vi "ex32.vi"(11 "Data":string) -> ()   [LabVIEW 2019]
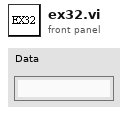
[diagram p1: front panel]
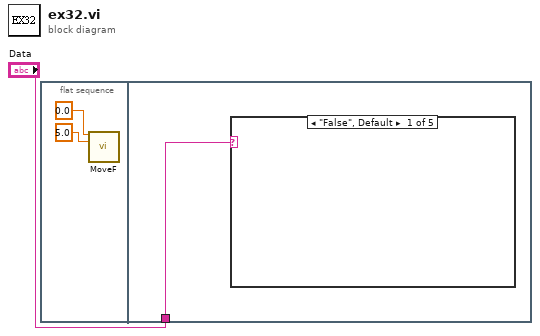
[diagram p0: block diagram]
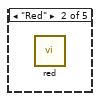
[diagram p2: hidden frame]
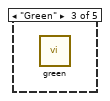
[diagram p3: hidden frame]
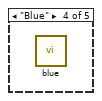
[diagram p4: hidden frame]
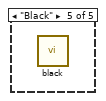
[diagram p5: hidden frame]
diagram:
  n1 = flat-sequence {
    tunnel: "Data" -> [w4]
    frame #0 {
      n2 = call "MoveF.vi"("X"=0.0, "Y"=5.0) -> ()  [unwired: 13 in, 1 out]
    }
    frame #1 {
      n3 = case shown="\"False\", Default" w4 {
        frame "False", Default {
        }
        frame "Red" {
          n4 = call "red.vi"() -> ()  [unwired: 11 in, 1 out]
        }
        frame "Green" {
          n5 = call "green.vi"() -> ()  [unwired: 11 in, 1 out]
        }
        frame "Blue" {
          n6 = call "blue.vi"() -> ()  [unwired: 11 in, 1 out]
        }
        frame "Black" {
          n7 = call "black.vi"() -> ()  [unwired: 11 in, 1 out]
        }
      }
    }
  }
